vi "Begin.vi"() -> (0 "error out":errorcluster)   [LabVIEW 2012]
doc: "Called before other user functions, this VI is expected to open initial I/O refnums, load in file data, and do all program initialization. Notice that the <B>error out</B> terminal is simply used for data flow. Wiring it to other structures or subVIs ensures that this VI runs first."
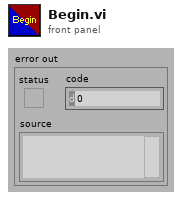
[diagram p1: front panel]
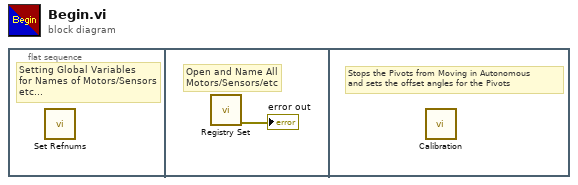
[diagram p0: block diagram]
diagram:
  n1 = flat-sequence {
    frame #0 {
      # "Setting Global Variables\nfor Names of Motors/Sensors\netc..."
      n2 = call "Set Refnums.vi"() -> ()  [unwired: 12 in]
    }
    frame #1 {
      # "Open and Name All\nMotors/Sensors/etc"
      n3 = call "Registry Set.vi"() -> ("error out"=→"error out":errorcluster)  [unwired: 11 in]
    }
    frame #2 {
      # "Stops the Pivots from Moving in Autonomous\nand sets the offset angles for the Pivots"
      n4 = call "Calibration.vi"() -> ()  [unwired: 12 in]
    }
  }
